vi "MotorScan.vi"() -> ()   [LabVIEW 2022 SP3]
panel:
  in  "Wait [s]":dbl format="%.3f"
  in  "Meas command":string="READ?"
  in  "InitSensor":string[](array[string])
  in  "InitMotor":string[](array[string])=["X 0", "Y 0", "Z 0"]
  in  "AutoInc":bool
  in  "filename":path
  in  "DataSel":u16(ring)=1 items=["D0", "D1", "D2", "D3"]
  in  "1D2D":bool
  out "1Dplot":cluster{"Axis1":dbl[], dbl[]}[](graph)=[{"Axis1"=[-50.0, -48.0, -46.0, -44.0, -42.0, -40.0, -38.0, -36.0, -34.0, -32.0, -30.0, -28.0, -26.0, -24.0, -22.0, -20.0, -18.0, -16.0, -14.0, -12.0, -10.0, -8.0, -6.0, -4.0, -2.0, 0.0, 2.0, 4.0, 6.0, 8.0, 10.0, 12.0, 14.0, 16.0, 18.0, 20.0, 22.0, 24.0, 26.0, 28.0, 30.0, 32.0, 34.0, 36.0, 38.0, 40.0, 42.0, 44.0, 46.0, 48.0, 50.0], [-2164.5, -2179.5, -2191.2, -2202.3, -2210.4, -2218.2, -2224.2, -2227.5, -2231.1, -2234.4, -2236.5, -2238.6, -2239.5, -2240.7, -2239.8, -2240.1, -2240.7, -2240.4, -2240.7, -2239.8, -2240.4, -2240.7, -2240.4, -2240.1, -2240.4, -2240.4, -2240.7, -2241.0, -2241.3, -2242.8, -2242.5, -2241.9, -2241.6, -2242.5, -2241.6, -2242.8, -2241.9, -2240.1, -2239.8, -2237.7, -2234.7, -2231.1, -2225.7, -2221.2, -2213.7, -2204.1, -2194.5, -2182.2, -2166.6, -2151.0, -2131.8]}, {"Axis1"=[-50.0, -48.0, -46.0, -44.0, -42.0, -40.0, -38.0, -36.0, -34.0, -32.0, -30.0, -28.0, -26.0, -24.0, -22.0, -20.0, -18.0, -16.0, -14.0, -12.0, -10.0, -8.0, -6.0, -4.0, -2.0, 0.0, 2.0, 4.0, 6.0, 8.0, 10.0, 12.0, 14.0, 16.0, 18.0, 20.0, 22.0, 24.0, 26.0, 28.0, 30.0, 32.0, 34.0, 36.0, 38.0, 40.0, 42.0, 44.0, 46.0, 48.0, 50.0], [-2150.4, -2164.2, -2178.0, -2190.3, -2200.8, -2208.6, -2215.8, -2220.6, -2225.7, -2228.7, -2231.7, -2234.1, -2235.0, -2236.2, -2238.0, -2238.6, -2239.8, -2238.9, -2239.8, -2239.2, -2239.5, -2239.5, -2240.1, -2238.9, -2240.4, -2239.5, -2239.2, -2240.1, -2240.1, -2240.1, -2240.1, -2239.2, -2238.9, -2238.6, -2238.0, -2237.4, -2236.2, -2235.9, -2232.3, -2229.9, -2226.0, -2221.8, -2215.8, -2209.2, -2202.6, -2191.8, -2180.4, -2167.2, -2151.6, -2133.0, -2110.8]}, {"Axis1"=[-50.0, -48.0, -46.0, -44.0, -42.0, -40.0, -38.0, -36.0, -34.0, -32.0, -30.0, -28.0, -26.0, -24.0, -22.0, -20.0, -18.0, -16.0, -14.0, -12.0, -10.0, -8.0, -6.0, -4.0, -2.0, 0.0, 2.0, 4.0, 6.0, 8.0, 10.0, 12.0, 14.0, 16.0, 18.0, 20.0, 22.0, 24.0, 26.0, 28.0, 30.0, 32.0, 34.0, 36.0, 38.0, 40.0, 42.0, 44.0, 46.0, 48.0, 50.0], [-2135.7, -2152.5, -2167.8, -2178.9, -2190.0, -2199.3, -2207.1, -2213.4, -2218.5, -2223.0, -2227.2, -2228.1, -2231.1, -2233.2, -2235.0, -2236.2, -2236.2, -2236.8, -2236.5, -2238.6, -2237.1, -2237.7, -2237.7, -2238.3, -2237.7, -2237.1, -2238.0, -2238.3, -2238.3, -2238.0, -2237.4, -2237.1, -2234.7, -2235.3, -2233.8, -2234.1, -2231.4, -2229.0, -2226.0, -2222.4, -2218.8, -2214.0, -2206.5, -2198.4, -2190.9, -2178.9, -2167.2, -2153.1, -2136.0, -2115.3, -2094.0]}, {"Axis1"=[-50.0, -48.0, -46.0, -44.0, -42.0, -40.0, -38.0, -36.0, -34.0, -32.0, -30.0, -28.0, -26.0, -24.0, -22.0, -20.0, -18.0, -16.0, -14.0, -12.0, -10.0, -8.0, -6.0, -4.0, -2.0, 0.0, 2.0, 4.0, 6.0, 8.0, 10.0, 12.0, 14.0, 16.0, 18.0, 20.0, 22.0, 24.0, 26.0, 28.0, 30.0, 32.0, 34.0, 36.0, 38.0, 40.0, 42.0, 44.0, 46.0, 48.0, 50.0], [-2124.9, -2143.8, -2158.5, -2170.8, -2182.2, -2193.3, -2201.4, -2208.0, -2212.8, -2216.7, -2222.1, -2225.1, -2227.8, -2229.3, -2231.7, -2233.2, -2233.5, -2232.3, -2233.8, -2234.7, -2234.1, -2235.6, -2234.7, -2235.3, -2235.0, -2235.9, -2235.9, -2234.4, -2235.3, -2234.1, -2233.8, -2233.5, -2232.9, -2232.6, -2231.7, -2229.6, -2228.1, -2225.7, -2222.1, -2217.0, -2212.8, -2207.7, -2199.6, -2191.5, -2183.1, -2171.1, -2156.4, -2141.4, -2123.4, -2103.3, -2080.2]}, {"Axis1"=[-50.0, -48.0, -46.0, -44.0, -42.0, -40.0, -38.0, -36.0, -34.0, -32.0, -30.0, -28.0, -26.0, -24.0, -22.0, -20.0, -18.0, -16.0, -14.0, -12.0, -10.0, -8.0, -6.0, -4.0, -2.0, 0.0, 2.0, 4.0, 6.0, 8.0, 10.0, 12.0, 14.0, 16.0, 18.0, 20.0, 22.0, 24.0, 26.0, 28.0, 30.0, 32.0, 34.0, 36.0, 38.0, 40.0, 42.0, 44.0, 46.0, 48.0, 50.0], [-2118.6, -2136.3, -2152.2, -2165.7, -2176.5, -2186.4, -2197.2, -2202.3, -2208.9, -2213.7, -2218.2, -2220.9, -2224.8, -2226.6, -2228.4, -2230.2, -2230.8, -2232.6, -2233.5, -2232.6, -2232.3, -2234.7, -2233.5, -2234.1, -2234.4, -2234.7, -2233.8, -2234.7, -2233.8, -2232.9, -2234.1, -2231.7, -2232.3, -2230.5, -2228.7, -2227.2, -2224.2, -2222.4, -2218.8, -2214.9, -2210.4, -2203.5, -2195.7, -2186.7, -2176.8, -2165.1, -2151.3, -2136.0, -2116.2, -2095.5, -2073.0]}, {"Axis1"=[-50.0, -48.0, -46.0, -44.0, -42.0, -40.0, -38.0, -36.0, -34.0, -32.0, -30.0, -28.0, -26.0, -24.0, -22.0, -20.0, -18.0, -16.0, -14.0, -12.0, -10.0, -8.0, -6.0, -4.0, -2.0, 0.0, 2.0, 4.0, 6.0, 8.0, 10.0, 12.0, 14.0, 16.0, 18.0, 20.0, 22.0, 24.0, 26.0, 28.0, 30.0, 32.0, 34.0, 36.0, 38.0, 40.0, 42.0, 44.0, 46.0, 48.0, 50.0], [-2116.5, -2134.2, -2151.0, -2163.9, -2175.9, -2185.8, -2194.8, -2201.7, -2206.8, -2213.1, -2217.6, -2221.5, -2223.0, -2225.1, -2228.4, -2229.0, -2231.1, -2230.8, -2232.0, -2232.0, -2232.0, -2232.3, -2232.6, -2233.2, -2233.2, -2234.4, -2233.2, -2233.8, -2232.9, -2232.3, -2231.1, -2231.1, -2230.2, -2229.0, -2226.6, -2224.8, -2223.3, -2220.6, -2216.7, -2212.8, -2206.8, -2199.6, -2192.7, -2184.0, -2173.2, -2160.9, -2147.4, -2130.9, -2111.7, -2091.3, -2067.0]}, {"Axis1"=[-50.0, -48.0, -46.0, -44.0, -42.0, -40.0, -38.0, -36.0, -34.0, -32.0, -30.0, -28.0, -26.0, -24.0, -22.0, -20.0, -18.0, -16.0, -14.0, -12.0, -10.0, -8.0, -6.0, -4.0, -2.0, 0.0, 2.0, 4.0, 6.0, 8.0, 10.0, 12.0, 14.0, 16.0, 18.0, 20.0, 22.0, 24.0, 26.0, 28.0, 30.0, 32.0, 34.0, 36.0, 38.0, 40.0, 42.0, 44.0, 46.0, 48.0, 50.0], [-2115.6, -2133.3, -2149.8, -2162.4, -2175.0, -2184.6, -2193.0, -2199.6, -2206.8, -2211.0, -2215.5, -2219.1, -2221.8, -2224.5, -2225.1, -2226.6, -2228.4, -2228.7, -2230.2, -2229.6, -2231.1, -2230.8, -2230.5, -2230.5, -2230.5, -2230.2, -2230.8, -2231.1, -2230.5, -2230.5, -2229.0, -2227.8, -2227.5, -2227.2, -2225.1, -2223.3, -2220.9, -2219.1, -2213.4, -2209.5, -2205.0, -2198.4, -2190.9, -2180.7, -2172.3, -2159.1, -2145.6, -2129.1, -2111.7, -2089.5, -2066.1]}, {"Axis1"=[-50.0, -48.0, -46.0, -44.0, -42.0, -40.0, -38.0, -36.0, -34.0, -32.0, -30.0, -28.0, -26.0, -24.0, -22.0, -20.0, -18.0, -16.0, -14.0, -12.0, -10.0, -8.0, -6.0, -4.0, -2.0, 0.0, 2.0, 4.0, 6.0, 8.0, 10.0, 12.0, 14.0, 16.0, 18.0, 20.0, 22.0, 24.0, 26.0, 28.0, 30.0, 32.0, 34.0, 36.0, 38.0, 40.0, 42.0, 44.0, 46.0, 48.0, 50.0], [-2118.6, -2136.0, -2151.6, -2163.6, -2175.6, -2184.9, -2192.4, -2201.1, -2205.6, -2211.0, -2215.5, -2218.8, -2221.2, -2224.2, -2225.1, -2226.0, -2227.2, -2228.1, -2228.1, -2229.3, -2228.7, -2230.2, -2229.6, -2229.9, -2230.5, -2229.3, -2229.6, -2230.5, -2229.0, -2229.0, -2228.4, -2227.8, -2227.5, -2226.3, -2224.8, -2222.7, -2220.3, -2217.9, -2213.1, -2209.8, -2204.7, -2197.8, -2191.8, -2182.2, -2170.8, -2160.6, -2146.8, -2130.9, -2113.5, -2092.8, -2069.7]}, {"Axis1"=[-50.0, -48.0, -46.0, -44.0, -42.0, -40.0, -38.0, -36.0, -34.0, -32.0, -30.0, -28.0, -26.0, -24.0, -22.0, -20.0, -18.0, -16.0, -14.0, -12.0, -10.0, -8.0, -6.0, -4.0, -2.0, 0.0, 2.0, 4.0, 6.0, 8.0, 10.0, 12.0, 14.0, 16.0, 18.0, 20.0, 22.0, 24.0, 26.0, 28.0, 30.0, 32.0, 34.0, 36.0, 38.0, 40.0, 42.0, 44.0, 46.0, 48.0, 50.0], [-2125.8, -2142.3, -2157.3, -2168.4, -2180.4, -2189.7, -2196.6, -2204.1, -2208.3, -2213.1, -2217.0, -2219.7, -2222.7, -2224.2, -2225.4, -2227.5, -2227.8, -2228.7, -2228.7, -2229.9, -2229.3, -2229.6, -2229.0, -2230.8, -2229.0, -2228.7, -2229.6, -2228.7, -2229.0, -2228.7, -2228.4, -2228.4, -2227.2, -2225.7, -2224.8, -2223.3, -2221.5, -2218.2, -2215.5, -2211.6, -2206.8, -2201.1, -2194.8, -2186.1, -2176.8, -2164.8, -2152.8, -2137.2, -2118.6, -2099.4, -2077.2]}, {"Axis1"=[-50.0, -48.0, -46.0, -44.0, -42.0, -40.0, -38.0, -36.0, -34.0, -32.0, -30.0, -28.0, -26.0, -24.0, -22.0, -20.0, -18.0, -16.0, -14.0, -12.0, -10.0, -8.0, -6.0, -4.0, -2.0, 0.0, 2.0, 4.0, 6.0, 8.0, 10.0, 12.0, 14.0, 16.0, 18.0, 20.0, 22.0, 24.0, 26.0, 28.0, 30.0, 32.0, 34.0, 36.0, 38.0, 40.0, 42.0, 44.0, 46.0, 48.0, 50.0], [-2135.7, -2151.9, -2164.5, -2176.2, -2186.1, -2195.4, -2202.0, -2208.3, -2213.7, -2217.0, -2220.3, -2222.7, -2224.2, -2226.6, -2227.8, -2228.4, -2227.8, -2229.6, -2229.3, -2229.6, -2229.0, -2228.7, -2229.9, -2229.0, -2229.3, -2229.9, -2229.0, -2229.0, -2229.0, -2228.7, -2227.8, -2229.0, -2227.8, -2228.7, -2226.3, -2224.8, -2223.6, -2220.9, -2218.5, -2215.5, -2210.1, -2206.2, -2199.6, -2191.8, -2183.1, -2172.9, -2160.6, -2145.6, -2128.8, -2109.0, -2088.0]}, {"Axis1"=[-50.0, -48.0, -46.0, -44.0, -42.0, -40.0, -38.0, -36.0, -34.0, -32.0, -30.0, -28.0, -26.0, -24.0, -22.0, -20.0, -18.0, -16.0, -14.0, -12.0, -10.0, -8.0, -6.0, -4.0, -2.0, 0.0, 2.0, 4.0, 6.0, 8.0, 10.0, 12.0, 14.0, 16.0, 18.0, 20.0, 22.0, 24.0, 26.0, 28.0, 30.0, 32.0, 34.0, 36.0, 38.0, 40.0, 42.0, 44.0, 46.0, 48.0, 50.0], [-2149.2, -2163.6, -2176.2, -2186.4, -2195.4, -2202.9, -2207.7, -2213.7, -2217.0, -2220.3, -2223.0, -2224.5, -2226.6, -2226.9, -2227.2, -2229.0, -2229.0, -2229.0, -2230.2, -2228.7, -2229.0, -2228.4, -2228.7, -2228.4, -2227.8, -2227.8, -2228.7, -2227.2, -2228.1, -2228.1, -2227.5, -2227.8, -2228.7, -2226.0, -2226.0, -2226.0, -2224.5, -2222.1, -2220.6, -2216.7, -2213.4, -2209.5, -2204.7, -2197.5, -2189.4, -2179.8, -2168.4, -2156.1, -2141.4, -2123.1, -2102.4]}]
  out "2Dplot":dbl[][](graph)=[[-2164.5, -2179.5, -2191.2, -2202.3, -2210.4, -2218.2, -2224.2, -2227.5, -2231.1, -2234.4, -2236.5, -2238.6, -2239.5, -2240.7, -2239.8, -2240.1, -2240.7, -2240.4, -2240.7, -2239.8, -2240.4, -2240.7, -2240.4, -2240.1, -2240.4, -2240.4, -2240.7, -2241.0, -2241.3, -2242.8, -2242.5, -2241.9, -2241.6, -2242.5, -2241.6, -2242.8, -2241.9, -2240.1, -2239.8, -2237.7, -2234.7, -2231.1, -2225.7, -2221.2, -2213.7, -2204.1, -2194.5, -2182.2, -2166.6, -2151.0, -2131.8], [-2150.4, -2164.2, -2178.0, -2190.3, -2200.8, -2208.6, -2215.8, -2220.6, -2225.7, -2228.7, -2231.7, -2234.1, -2235.0, -2236.2, -2238.0, -2238.6, -2239.8, -2238.9, -2239.8, -2239.2, -2239.5, -2239.5, -2240.1, -2238.9, -2240.4, -2239.5, -2239.2, -2240.1, -2240.1, -2240.1, -2240.1, -2239.2, -2238.9, -2238.6, -2238.0, -2237.4, -2236.2, -2235.9, -2232.3, -2229.9, -2226.0, -2221.8, -2215.8, -2209.2, -2202.6, -2191.8, -2180.4, -2167.2, -2151.6, -2133.0, -2110.8], [-2135.7, -2152.5, -2167.8, -2178.9, -2190.0, -2199.3, -2207.1, -2213.4, -2218.5, -2223.0, -2227.2, -2228.1, -2231.1, -2233.2, -2235.0, -2236.2, -2236.2, -2236.8, -2236.5, -2238.6, -2237.1, -2237.7, -2237.7, -2238.3, -2237.7, -2237.1, -2238.0, -2238.3, -2238.3, -2238.0, -2237.4, -2237.1, -2234.7, -2235.3, -2233.8, -2234.1, -2231.4, -2229.0, -2226.0, -2222.4, -2218.8, -2214.0, -2206.5, -2198.4, -2190.9, -2178.9, -2167.2, -2153.1, -2136.0, -2115.3, -2094.0], [-2124.9, -2143.8, -2158.5, -2170.8, -2182.2, -2193.3, -2201.4, -2208.0, -2212.8, -2216.7, -2222.1, -2225.1, -2227.8, -2229.3, -2231.7, -2233.2, -2233.5, -2232.3, -2233.8, -2234.7, -2234.1, -2235.6, -2234.7, -2235.3, -2235.0, -2235.9, -2235.9, -2234.4, -2235.3, -2234.1, -2233.8, -2233.5, -2232.9, -2232.6, -2231.7, -2229.6, -2228.1, -2225.7, -2222.1, -2217.0, -2212.8, -2207.7, -2199.6, -2191.5, -2183.1, -2171.1, -2156.4, -2141.4, -2123.4, -2103.3, -2080.2], [-2118.6, -2136.3, -2152.2, -2165.7, -2176.5, -2186.4, -2197.2, -2202.3, -2208.9, -2213.7, -2218.2, -2220.9, -2224.8, -2226.6, -2228.4, -2230.2, -2230.8, -2232.6, -2233.5, -2232.6, -2232.3, -2234.7, -2233.5, -2234.1, -2234.4, -2234.7, -2233.8, -2234.7, -2233.8, -2232.9, -2234.1, -2231.7, -2232.3, -2230.5, -2228.7, -2227.2, -2224.2, -2222.4, -2218.8, -2214.9, -2210.4, -2203.5, -2195.7, -2186.7, -2176.8, -2165.1, -2151.3, -2136.0, -2116.2, -2095.5, -2073.0], [-2116.5, -2134.2, -2151.0, -2163.9, -2175.9, -2185.8, -2194.8, -2201.7, -2206.8, -2213.1, -2217.6, -2221.5, -2223.0, -2225.1, -2228.4, -2229.0, -2231.1, -2230.8, -2232.0, -2232.0, -2232.0, -2232.3, -2232.6, -2233.2, -2233.2, -2234.4, -2233.2, -2233.8, -2232.9, -2232.3, -2231.1, -2231.1, -2230.2, -2229.0, -2226.6, -2224.8, -2223.3, -2220.6, -2216.7, -2212.8, -2206.8, -2199.6, -2192.7, -2184.0, -2173.2, -2160.9, -2147.4, -2130.9, -2111.7, -2091.3, -2067.0], [-2115.6, -2133.3, -2149.8, -2162.4, -2175.0, -2184.6, -2193.0, -2199.6, -2206.8, -2211.0, -2215.5, -2219.1, -2221.8, -2224.5, -2225.1, -2226.6, -2228.4, -2228.7, -2230.2, -2229.6, -2231.1, -2230.8, -2230.5, -2230.5, -2230.5, -2230.2, -2230.8, -2231.1, -2230.5, -2230.5, -2229.0, -2227.8, -2227.5, -2227.2, -2225.1, -2223.3, -2220.9, -2219.1, -2213.4, -2209.5, -2205.0, -2198.4, -2190.9, -2180.7, -2172.3, -2159.1, -2145.6, -2129.1, -2111.7, -2089.5, -2066.1], [-2118.6, -2136.0, -2151.6, -2163.6, -2175.6, -2184.9, -2192.4, -2201.1, -2205.6, -2211.0, -2215.5, -2218.8, -2221.2, -2224.2, -2225.1, -2226.0, -2227.2, -2228.1, -2228.1, -2229.3, -2228.7, -2230.2, -2229.6, -2229.9, -2230.5, -2229.3, -2229.6, -2230.5, -2229.0, -2229.0, -2228.4, -2227.8, -2227.5, -2226.3, -2224.8, -2222.7, -2220.3, -2217.9, -2213.1, -2209.8, -2204.7, -2197.8, -2191.8, -2182.2, -2170.8, -2160.6, -2146.8, -2130.9, -2113.5, -2092.8, -2069.7], [-2125.8, -2142.3, -2157.3, -2168.4, -2180.4, -2189.7, -2196.6, -2204.1, -2208.3, -2213.1, -2217.0, -2219.7, -2222.7, -2224.2, -2225.4, -2227.5, -2227.8, -2228.7, -2228.7, -2229.9, -2229.3, -2229.6, -2229.0, -2230.8, -2229.0, -2228.7, -2229.6, -2228.7, -2229.0, -2228.7, -2228.4, -2228.4, -2227.2, -2225.7, -2224.8, -2223.3, -2221.5, -2218.2, -2215.5, -2211.6, -2206.8, -2201.1, -2194.8, -2186.1, -2176.8, -2164.8, -2152.8, -2137.2, -2118.6, -2099.4, -2077.2], [-2135.7, -2151.9, -2164.5, -2176.2, -2186.1, -2195.4, -2202.0, -2208.3, -2213.7, -2217.0, -2220.3, -2222.7, -2224.2, -2226.6, -2227.8, -2228.4, -2227.8, -2229.6, -2229.3, -2229.6, -2229.0, -2228.7, -2229.9, -2229.0, -2229.3, -2229.9, -2229.0, -2229.0, -2229.0, -2228.7, -2227.8, -2229.0, -2227.8, -2228.7, -2226.3, -2224.8, -2223.6, -2220.9, -2218.5, -2215.5, -2210.1, -2206.2, -2199.6, -2191.8, -2183.1, -2172.9, -2160.6, -2145.6, -2128.8, -2109.0, -2088.0], [-2149.2, -2163.6, -2176.2, -2186.4, -2195.4, -2202.9, -2207.7, -2213.7, -2217.0, -2220.3, -2223.0, -2224.5, -2226.6, -2226.9, -2227.2, -2229.0, -2229.0, -2229.0, -2230.2, -2228.7, -2229.0, -2228.4, -2228.7, -2228.4, -2227.8, -2227.8, -2228.7, -2227.2, -2228.1, -2228.1, -2227.5, -2227.8, -2228.7, -2226.0, -2226.0, -2226.0, -2224.5, -2222.1, -2220.6, -2216.7, -2213.4, -2209.5, -2204.7, -2197.5, -2189.4, -2179.8, -2168.4, -2156.1, -2141.4, -2123.1, -2102.4]]
  in  "Abort":bool
  out "Moving":bool
  in  "Sensor VISA":refnum<visa-resource-name>="COM6"
  out "Act2 [mm]":dbl=-10.0 format="%.3p"
  out "Act1 [mm]":dbl=-50.0 format="%.3p"
  in  "ustep2":u16(ring)=4 items=["full"=1, "1/2"=2, "1/4"=4, "1/8"=8, "1/16"=16]
  in  "ustep1":u16(ring)=4 items=["full"=1, "1/2"=2, "1/4"=4, "1/8"=8, "1/16"=16]
  in  "Axis2":u16(ring)=1 items=["X", "Y", "Z"]
  in  "#pts2":u32=11
  in  "Start2 [mm]":dbl=-10.0 format="%.3p"
  in  "Stop2 [mm]":dbl=10.0 format="%.3p"
  in  "#pts1":u32=51
  in  "Stop1 [mm]":dbl=50.0 format="%.3p"
  in  "Start1 [mm]":dbl=-50.0 format="%.3p"
  in  "Axis1":u16(ring) items=["X", "Y", "Z"]
  in  "Motor VISA":refnum<visa-resource-name>="COM4"
  # "Motor Scan"
  # "Measurement Data"
  # "1D"
  # "2D"
  # "* NB la posizione di partenza viene impostata a (0,0,0)\n* Abort blocca tutto e riporta al punto di partenza"
  # "Sweep setup"
  # "Save on file"
  # "Filename\nautoincrement?"
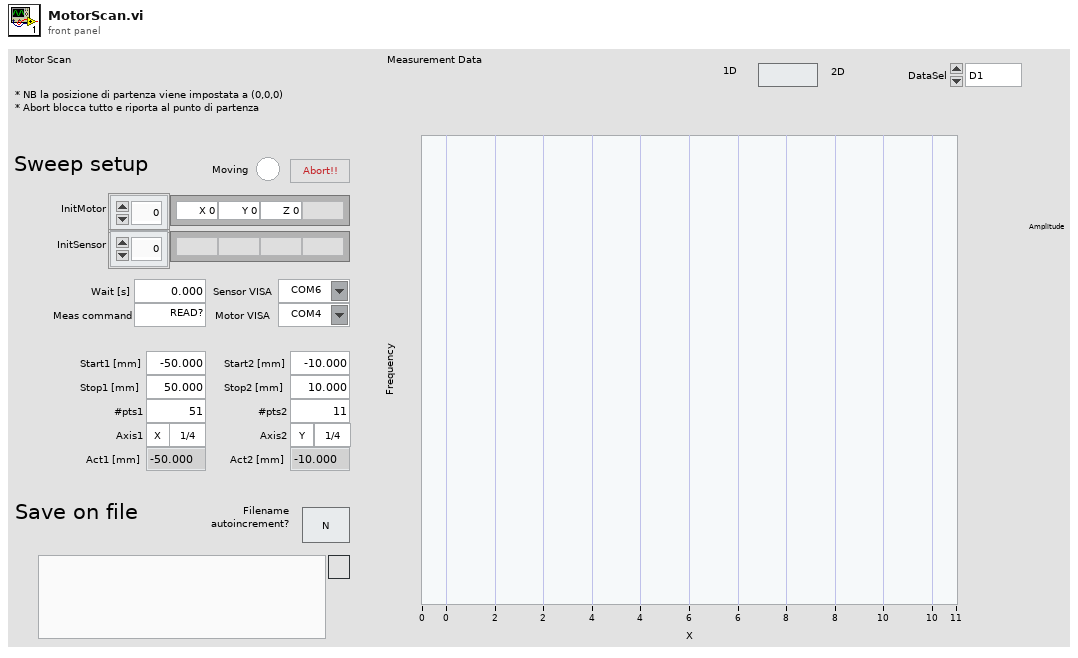
[diagram p1: front panel]
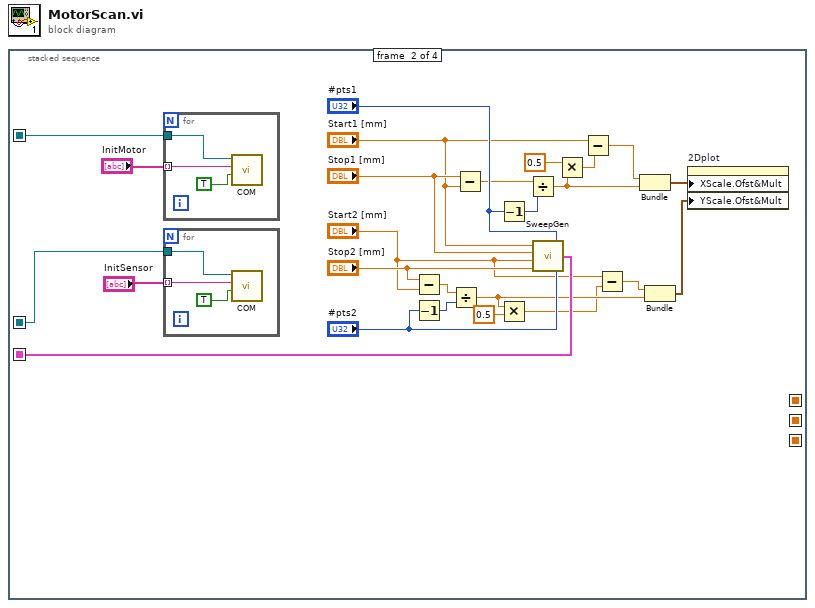
[diagram p0: block diagram]
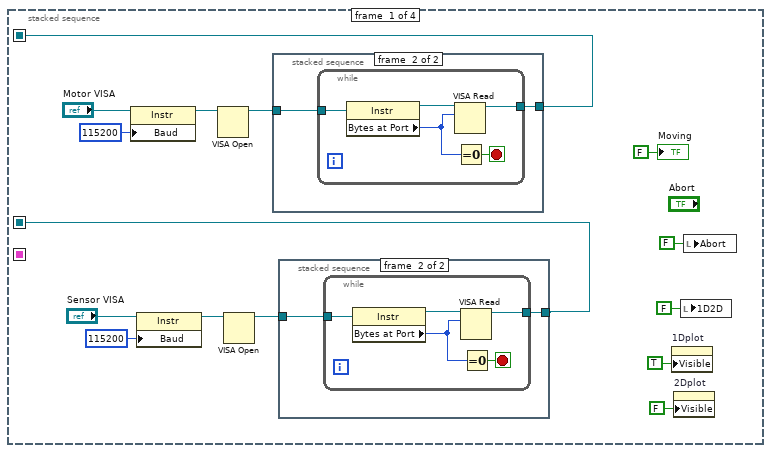
[diagram p2: hidden frame]
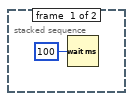
[diagram p3: hidden frame]
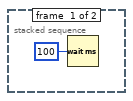
[diagram p4: hidden frame]
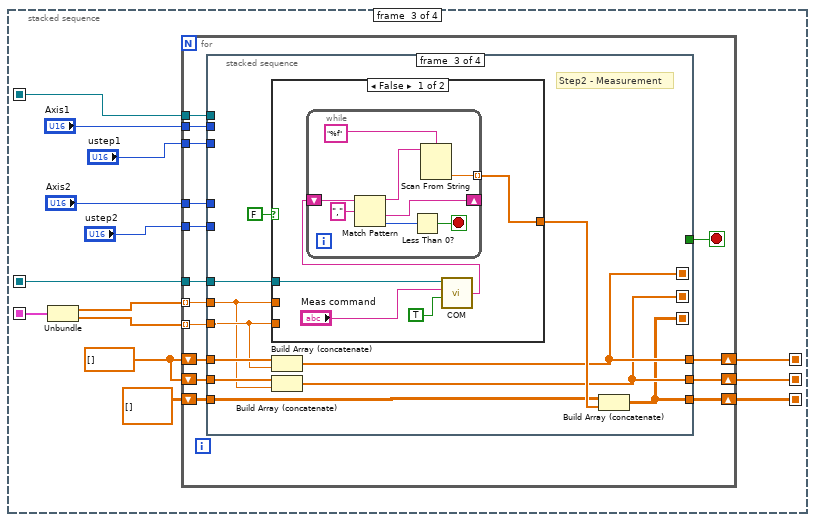
[diagram p5: hidden frame]
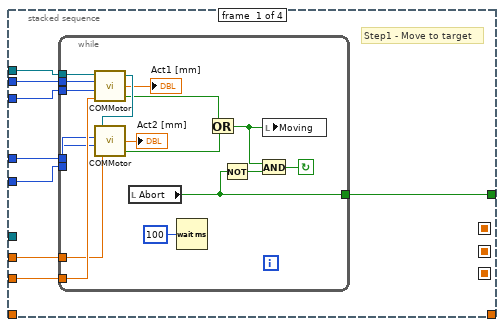
[diagram p6: hidden frame]
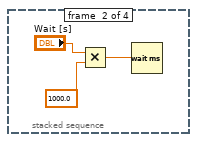
[diagram p7: hidden frame]
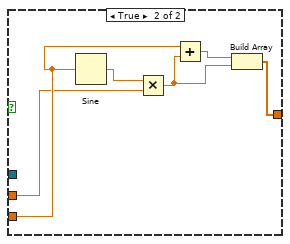
[diagram p8: hidden frame]
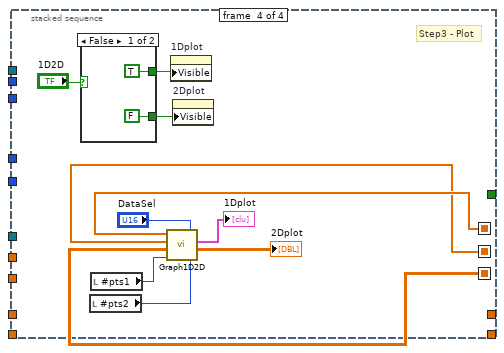
[diagram p9: hidden frame]
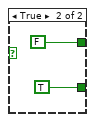
[diagram p10: hidden frame]
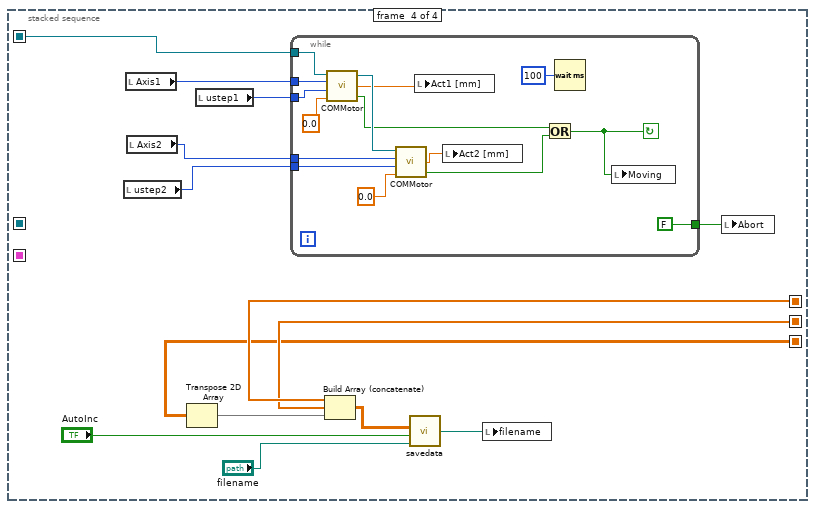
[diagram p11: hidden frame]
diagram:
  n1 = stacked-sequence {
    seq-local: [w11 _ _ _] -> [_ w56 w76 w178]
    seq-local: [_ w54 _ _] -> [_ _ w71 _]
    seq-local: [w4 _ _ _] -> [_ w52 w68 _]
    seq-local: [_ _ w65 _] -> [_ _ _ w169]
    seq-local: [_ _ w64 _] -> [_ _ _ w168]
    seq-local: [_ _ w63 _] -> [_ _ _ w165]
    frame #0 {
      n2 = property class="Instr"(reference="Motor VISA", "Baud"=u32 115200 ("Serial Settings:Baud Rate")) -> (reference out=w13:refnum<visa-resource-name>)  [unwired: 1 in, 1 out]
      n3 = property class="Instr"(reference="Sensor VISA", "Baud"=u32 115200 ("Serial Settings:Baud Rate")) -> (reference out=w7:refnum<visa-resource-name>)  [unwired: 1 in, 1 out]
      n4 = VISA Open(VISA resource name=w13) -> (VISA resource name=w12:refnum<visa-resource-name>)  [unwired: 4 in, 1 out]
      n5 = VISA Open(VISA resource name=w7) -> (VISA resource name=w6:refnum<visa-resource-name>)  [unwired: 4 in, 1 out]
      n6 = stacked-sequence {
        tunnel: w12 -> [_ w26]
        tunnel: [_ w25] -> w11
        frame #0 {
          n7 = Wait (ms)(milliseconds to wait=u32 100) -> ()  [unwired: 1 out]
        }
        frame #1 {
          n8 = while {
            tunnel: w26 -> [w31]
            tunnel: [w27] -> w25
            stop <- w28 stop-if-true
            n9 = property class="Instr"(reference=w31) -> (reference out=w30:refnum<visa-resource-name>, "Bytes at Port"=w29:u32)  [unwired: 1 in, 1 out]
            n10 = VISA Read(VISA resource name=w30, byte count=w29) -> (VISA resource name out=w27:refnum<visa-resource-name>)  [unwired: 1 in, 3 out]
            n11 = Equal To 0?(x=w29) -> (x = 0?=w28:bool)
          }
        }
      }
      n12 = stacked-sequence {
        tunnel: w6 -> [_ w18]
        tunnel: [_ w17] -> w4
        frame #0 {
          n13 = Wait (ms)(milliseconds to wait=u32 100) -> ()  [unwired: 1 out]
        }
        frame #1 {
          n14 = while {
            tunnel: w18 -> [w23]
            tunnel: [w19] -> w17
            stop <- w20 stop-if-true
            n15 = property class="Instr"(reference=w23) -> (reference out=w22:refnum<visa-resource-name>, "Bytes at Port"=w21:u32)  [unwired: 1 in, 1 out]
            n16 = VISA Read(VISA resource name=w22, byte count=w21) -> (VISA resource name out=w19:refnum<visa-resource-name>)  [unwired: 1 in, 3 out]
            n17 = Equal To 0?(x=w21) -> (x = 0?=w20:bool)
          }
        }
      }
      n18 = property on="1Dplot" class="XYGraph (strict)"("Visible"=TRUE) -> ()  [unwired: 2 in, 2 out]
      n19 = property on="2Dplot" class="IntGraph (strict)"("Visible"=FALSE) -> ()  [unwired: 2 in, 2 out]
      n20 = local write "1D2D"(FALSE ("1D2D")) -> ()
      n21 = local write "Abort"(FALSE ("Abort")) -> ()
      "Moving" <- FALSE ("Moving")
    }
    frame #1 {
      n22 = for {
        tunnel: w56 -> [w61]
        tunnel: "InitMotor" -> [w60] mode=indexing
        n23 = call "COM.vi"("Write?"=TRUE, "command"=w60, "VISA in"=w61) -> ()  [unwired: 1 in, 3 out]
      }
      n24 = for {
        tunnel: w52 -> [w58]
        tunnel: "InitSensor" -> [w57] mode=indexing
        n25 = call "COM.vi"("Write?"=TRUE, "command"=w57, "VISA in"=w58) -> ()  [unwired: 1 in, 3 out]
      }
      n26 = Subtract(x="Stop2 [mm]", y="Start2 [mm]") -> (x-y=w49:dbl)
      n27 = Decrement(x="#pts2") -> (x-1=w48:u32)
      n28 = Divide(x=w49, y=w48) -> (x/y=w34:dbl)
      n29 = Subtract(x="Stop1 [mm]", y="Start1 [mm]") -> (x-y=w45:dbl)
      n30 = Decrement(x="#pts1") -> (x-1=w44:u32)
      n31 = Multiply(x=w34, y=0.5 ("x")) -> (x*y=w32:dbl)
      n32 = Divide(x=w45, y=w44) -> (x/y=w41:dbl)
      n33 = call "SweepGen.vi"("#pts2"="#pts2", "#pts1"="#pts1", "Stop2"="Stop2 [mm]", "Start2"="Start2 [mm]", "Stop1"="Stop1 [mm]", "Start1"="Start1 [mm]") -> ("Sweep"=w54:cluster{dbl[], dbl[]})
      n34 = Multiply(x=0.5, y=w41) -> (x*y=w38:dbl)
      n35 = Subtract(x="Start1 [mm]", y=w38) -> (x-y=w37:dbl)
      n36 = Subtract(x="Start2 [mm]", y=w32) -> (x-y=w35:dbl)
      n37 = Bundle(w37, w41) -> (w43:cluster{dbl, dbl})  [unwired: 1 in]
      n38 = Bundle(w35, w34) -> (w42:cluster{dbl, dbl})  [unwired: 1 in]
      n39 = property on="2Dplot" class="IntGraph (strict)"("XScale.Ofst&Mult"=w43, "YScale.Ofst&Mult"=w42) -> ()  [unwired: 2 in, 2 out]
    }
    frame #2 {
      w67 = dbl[] []
      n40 = Unbundle(w71) -> (w70:dbl[], w69:dbl[])
      n41 = for {
        tunnel: w76 -> [w91]
        tunnel: "Axis1" -> [w90]
        tunnel: "ustep1" -> [w89]
        tunnel: "Axis2" -> [w88]
        tunnel: "ustep2" -> [w87]
        tunnel: w70 -> [w86] mode=indexing
        tunnel: w69 -> [w85] mode=indexing
        tunnel: w68 -> [w83]
        shift-right: [w81] -> w65
        shift-left: w67 -> [w82]
        shift-right: [w79] -> w64
        shift-left: w67 -> [w80]
        shift-right: [w78] -> w63
        shift-left: dbl[][] [] -> [w77]
        stop <- w84 stop-if-true
        n42 = stacked-sequence {
          seq-local: [_ _ w124 _] -> [_ _ _ w155]
          seq-local: [_ _ w125 _] -> [_ _ _ w156]
          seq-local: [_ _ w126 _] -> [_ _ _ w157]
          tunnel: w91 -> [w99 _ _ _]
          tunnel: w90 -> [w98 _ _ _]
          tunnel: w89 -> [w97 _ _ _]
          tunnel: w88 -> [w96 _ _ _]
          tunnel: w87 -> [w95 _ _ _]
          tunnel: w86 -> [w94 _ w122 _]
          tunnel: w85 -> [w93 _ w123 _]
          tunnel: [w92 _ _ _] -> w84
          tunnel: w83 -> [_ _ w120 _]
          tunnel: w82 -> [_ _ w130 _]
          tunnel: [_ _ w126 _] -> w81
          tunnel: w80 -> [_ _ w129 _]
          tunnel: [_ _ w125 _] -> w79
          tunnel: [_ _ w124 _] -> w78
          tunnel: w77 -> [_ _ w127 _]
          frame #0 {
            # "Step1 - Move to target"
            n43 = while {
              tunnel: w99 -> [w116]
              tunnel: w98 -> [w115]
              tunnel: w97 -> [w114]
              tunnel: w93 -> [w113]
              tunnel: w96 -> [w111]
              tunnel: w95 -> [w110]
              tunnel: w94 -> [w109]
              tunnel: [w100] -> w92
              stop <- w103 continue-if-true
              n44 = call "COMMotor.vi"("Target [mm]"=w113, "ustep"=w114, "axis"=w115, "VISA in"=w116) -> ("Moving"=w106:bool, "Position [mm]"=→"Act1 [mm]":dbl, "VISA out"=w112:refnum<visa-resource-name>)
              n45 = call "COMMotor.vi"("Target [mm]"=w109, "ustep"=w110, "axis"=w111, "VISA in"=w112) -> ("Moving"=w105:bool, "Position [mm]"=→"Act2 [mm]":dbl)  [unwired: 1 out]
              n46 = local read "Abort"() -> (w100:bool)
              n47 = Wait (ms)(milliseconds to wait=u32 100) -> ()  [unwired: 1 out]
              n48 = Or(x=w106, y=w105) -> (x .or. y?=w101:bool)
              n49 = Not(x=w100) -> (.not. x?=w102:bool)
              n50 = And(x=w101, y=w102) -> (x .and. y?=w103:bool)
              n51 = local write "Moving"(w101) -> ()
            }
          }
          frame #1 {
            n52 = Multiply(x="Wait [s]", y=1000.0) -> (x*y=w117:dbl)
            n53 = Wait (ms)(milliseconds to wait=w117) -> ()  [unwired: 1 out]
          }
          frame #2 {
            # "Step2 - Measurement"
            n54 = case shown="False" FALSE {
              tunnel: [w133 w146] -> w128
              tunnel: w123 -> [_ w145]
              tunnel: w122 -> [_ w144]
              tunnel: w120 -> [w135 _]
              frame False {
                n55 = call "COM.vi"("Write?"=TRUE, "command"="Meas command", "VISA in"=w135) -> ("reply"=w134:string)  [unwired: 1 in, 2 out]
                n56 = while {
                  shift-right: [w142] -> _
                  shift-left: w134 -> [w143]
                  tunnel: [w140] -> w133 mode=indexing
                  stop <- w138 stop-if-true
                  n57 = Match Pattern(string=w143, regular expression=",") -> (before substring=w141:string, after substring=w142:string, offset past match=w137:i32)  [unwired: 1 in, 1 out]
                  n58 = Less Than 0?(x=w137) -> (x < 0?=w138:bool)
                  n59 = Scan From String(format string="%f", input string=w141) -> (output 1=w140:dbl)  [unwired: 3 in, 3 out]
                }
              }
              frame True {
                n60 = Sine(x=w145) -> (sin(x)=w149:dbl)
                n61 = Multiply(x=w149, y=w144) -> (x*y=w147:dbl)
                n62 = Add(x=w145, y=w147) -> (x+y=w148:dbl)
                n63 = Build Array(w148, w147) -> (w146:dbl[])
              }
            }
            n64 = Build Array (concatenate)(w130, w123) -> (w126:dbl[])
            n65 = Build Array (concatenate)(w129, w122) -> (w125:dbl[])
            n66 = Build Array (concatenate)(w127, w128) -> (w124:dbl[][])
          }
          frame #3 {
            # "Step3 - Plot"
            n67 = case shown="False" "1D2D" {
              tunnel: [FALSE ("Visible") TRUE ("Visible")] -> w159
              tunnel: [TRUE ("Visible") FALSE ("Visible")] -> w158
              frame False {
              }
              frame True {
              }
            }
            n68 = local read "#pts2"() -> (w153:u32)
            n69 = local read "#pts1"() -> (w154:u32)
            n70 = call "Graph1D2D.vi"("#pts2"=w153, "DataSel"="DataSel", "#pts1"=w154, "Data"=w155, "Axis2"=w156, "Axis1"=w157) -> ("2Dplot"=→"2Dplot":dbl[][], "1Dplot"=→"1Dplot":cluster{"Axis1":dbl[], dbl[]}[])
            n71 = property on="1Dplot" class="XYGraph (strict)"("Visible"=w158) -> ()  [unwired: 2 in, 2 out]
            n72 = property on="2Dplot" class="IntGraph (strict)"("Visible"=w159) -> ()  [unwired: 2 in, 2 out]
          }
        }
      }
    }
    frame #3 {
      n73 = local read "ustep2"() -> (w174:u16)
      n74 = local read "Axis1"() -> (w177:u16)
      n75 = local read "Axis2"() -> (w175:u16)
      n76 = Transpose 2D Array(2D array=w165) -> (transposed array=w166:dbl[][])
      n77 = local read "ustep1"() -> (w176:u16)
      n78 = while {
        tunnel: w178 -> [w193]
        tunnel: w177 -> [w192]
        tunnel: w176 -> [w191]
        tunnel: w175 -> [w189]
        tunnel: w174 -> [w188]
        tunnel: [FALSE ("Abort")] -> w173
        stop <- w180 continue-if-true
        n79 = call "COMMotor.vi"("Target [mm]"=0.0, "ustep"=w191, "axis"=w192, "VISA in"=w193) -> ("Moving"=w187:bool, "Position [mm]"=w182:dbl, "VISA out"=w190:refnum<visa-resource-name>)
        n80 = call "COMMotor.vi"("Target [mm]"=0.0, "ustep"=w188, "axis"=w189, "VISA in"=w190) -> ("Moving"=w186:bool, "Position [mm]"=w181:dbl)  [unwired: 1 out]
        n81 = local write "Act1 [mm]"(w182) -> ()
        n82 = local write "Act2 [mm]"(w181) -> ()
        n83 = Or(x=w187, y=w186) -> (x .or. y?=w180:bool)
        n84 = Wait (ms)(milliseconds to wait=u32 100) -> ()  [unwired: 1 out]
        n85 = local write "Moving"(w180) -> ()
      }
      n86 = Build Array (concatenate)(w169, w168, w166) -> (w167:dbl[][])
      n87 = call "savedata.vi"("fnin"="filename", "Autoinc?"="AutoInc", "2Darray"=w167) -> ("fnout"=w172:path)  [unwired: 1 in]
      n88 = local write "filename"(w172) -> ()
      n89 = local write "Abort"(w173) -> ()
    }
  }
